vi "ex_subExcelFileWrite.vi"(8 "error in (no error)":errorcluster, 9 "configurations":T1={"new_file"=FALSE, "multi_file"=FALSE, "Enable"=TRUE, "File Dialog"=FALSE, "x_columns"=enum."none", "Ask each iteration"=FALSE, "overwrite_mode"=enum."overwrite", "setting"={"new_file_mode"=1, "Width"=2, "time_format_string"="%Y-%m-%d", "fixed_width"=TRUE, "overwrite_mode_multi"=1, "serno_digits"=3}, "new file options"={{"new_file_iter"=FALSE, "new_file_#iter"=0}, {"new_file_samples"=FALSE, "new_file_#samples"=0}, {"new_file_size"=FALSE, "new_file_max_size"=0}, {"new_file_elaps_time"=FALSE, "seconds"=0}, {"new_file_daily"=FALSE, "new_file_timeofday"=0}}, "reset"=FALSE, "Flush"=FALSE, "Static File Path in"=path "", "timestamp"={"absolute time"=TRUE, "Timestamp format"=""}} {"setting"."new_file_mode" items=["Date & Time", "Serial No.", "Both"]}, 10 "File path":path, 11 "Signals":dynamicdata(waveform)) -> (0 "error out":errorcluster, 2 "Saving Data":bool, 3 "Filename out":path)   [LabVIEW 2020]
uses:
  <vilib>/express/express output/ExFileWriteBlock.llb/ex_ExcelAllConfig.ctl
  <vilib>/express/express output/ExFileWriteBlock.llb/ex_NewFileOptions.ctl
  <vilib>/express/express output/ExFileWriteBlock.llb/ex_ExcelAdvancedConfig.ctl
  <vilib>/express/express shared/ExFile.llb/ex_userDefProperty.ctl
  <vilib>/express/express shared/ex_EditUserDefinedProperties/usiDataType.ctl
  <vilib>/express/express shared/ExFile.llb/ex_propertySource.ctl
  <vilib>/express/express shared/NI_ExcelFile/Ctrls/ExcelRefnum.ctl
  <vilib>/express/express shared/NI_ExcelFile/Ctrls/MainData.ctl
  <vilib>/express/express shared/NI_ExcelFile/Ctrls/StreamMode.ctl
  <vilib>/express/express shared/NI_ExcelFile/Ctrls/TimeColumnMode.ctl
  <vilib>/express/express shared/NI_ExcelFile/Ctrls/FileAttribute.ctl
  <vilib>/express/express shared/NI_ExcelFile/Ctrls/Columns.ctl
  <vilib>/express/express shared/NI_ExcelFile/Ctrls/ColumnInfo.ctl
  <vilib>/express/express shared/NI_ExcelFile/Ctrls/DataType.ctl
  <vilib>/express/express shared/NI_ExcelFile/Ctrls/wd_recordInfo.ctl
  <vilib>/express/express shared/NI_ExcelFile/Ctrls/disk_TemplateFile.ctl
  <vilib>/express/express shared/NI_ExcelFile/Ctrls/meta_file.ctl
  <vilib>/express/express shared/NI_ExcelFile/Ctrls/meta_Block.ctl
  <vilib>/express/express shared/NI_ExcelFile/Ctrls/meta_BlockType.ctl
  <vilib>/express/express shared/NI_ExcelFile/NI_ExcelFile.lvlib
panel:
  out "previous path":path
  in  "1st":bool
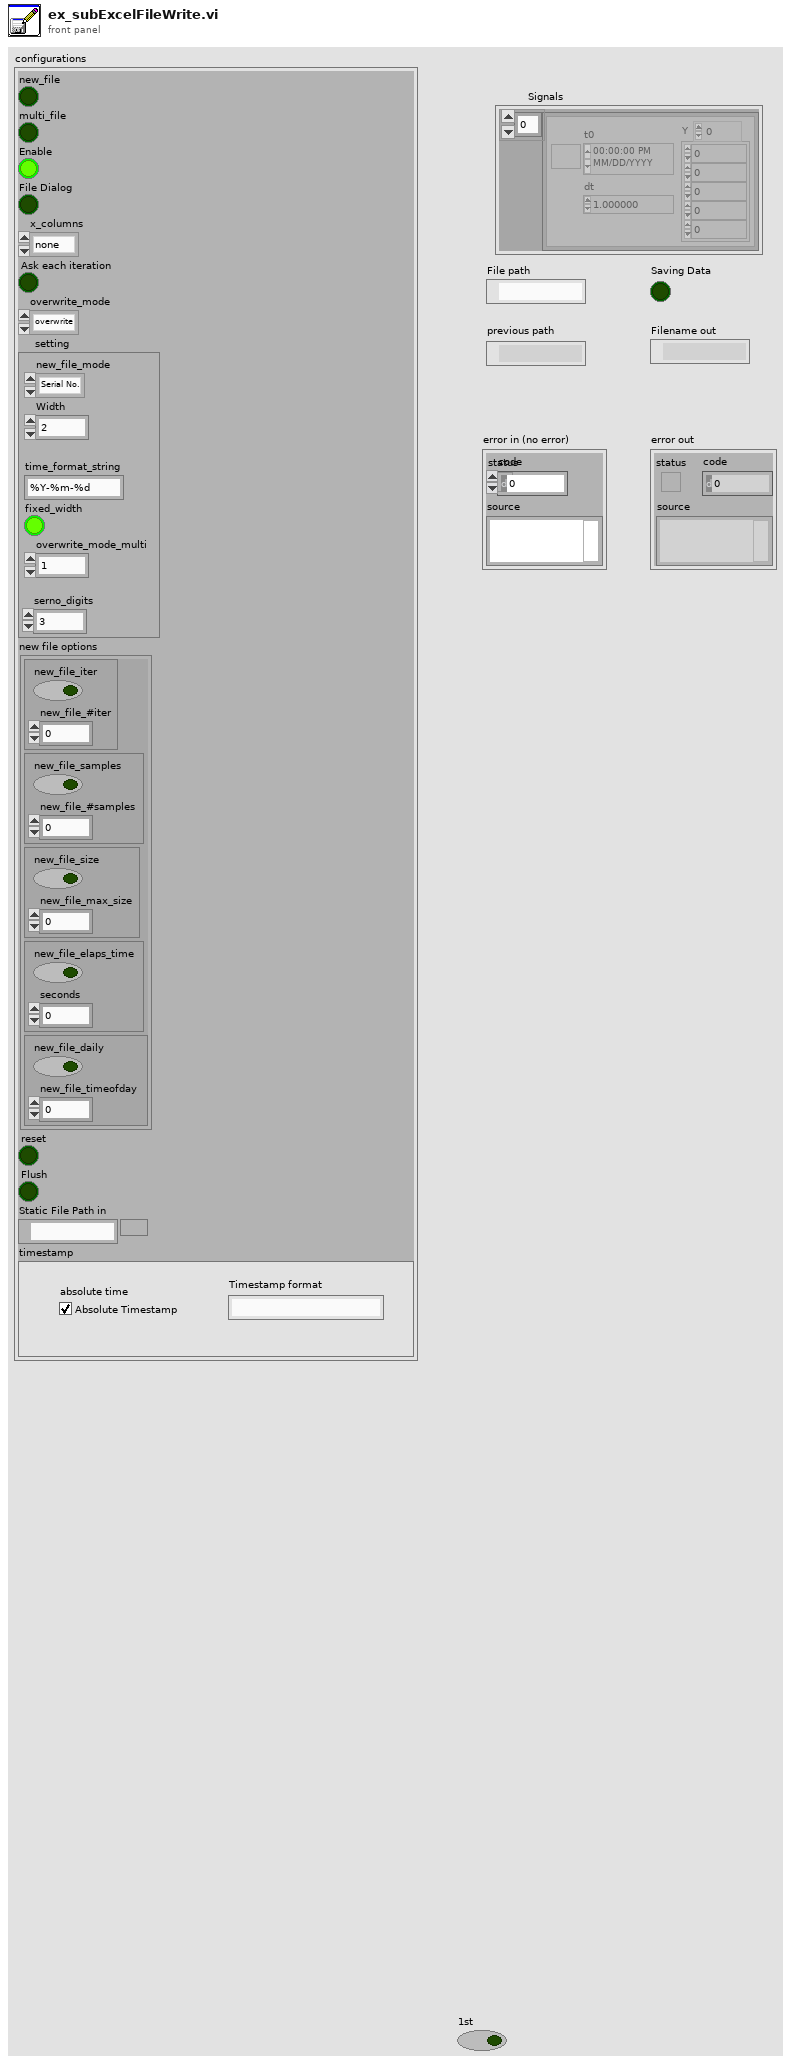
[diagram p1: front panel]
types:
  T1 = typedef "ex_ExcelAllConfig.ctl" = cluster{"new_file":bool, "multi_file":bool, "Enable":bool, "File Dialog":bool, "x_columns":enum32{"none", "one", "multiple"}, "Ask each iteration":bool, "overwrite_mode":enum32{"overwrite", "overwrite & backup", "append", "next avail"}, "setting":cluster{"new_file_mode":u16, "Width":i32, "time_format_string":string, "fixed_width":bool, "overwrite_mode_multi":i32, "serno_digits":i32}, "new file options":T2, "reset":bool, "Flush":bool, "Static File Path in":path, "timestamp":T3}
  T2 = typedef "ex_NewFileOptions.ctl" = cluster{cluster{"new_file_iter":bool, "new_file_#iter":i32}, cluster{"new_file_samples":bool, "new_file_#samples":i32}, cluster{"new_file_size":bool, "new_file_max_size":i32}, cluster{"new_file_elaps_time":bool, "seconds":i32}, cluster{"new_file_daily":bool, "new_file_timeofday":i32}}
  T3 = typedef "ex_ExcelAdvancedConfig.ctl" = cluster{"absolute time":bool, "Timestamp format":string}
  T4 = typedef "ex_userDefProperty.ctl" = cluster{"Name":string, "Object type":string, "usiDataType":T5, "propertySourceType":T6, "propertySource":string, "Value":variant, "ID":i32, "use def name":bool, "Source":string, "Built-in Prop":bool, "Attribute Type Enum":string[]}
  T5 = typedef "usiDataType.ctl" = enum16{"eNoTypeUsi", "eInt8Usi", "eInt16Usi", "eInt32Usi", "eInt64Usi", "eUInt8Usi", "eUInt16Usi", "eUInt32Usi", "eUInt64Usi", "eFloat32Usi", "eFloat64Usi", "- 0", "- 1", "- 2", "- 3", "- 4", "- 5", "- 6", "- 7", "- 8", "- 9", "eString8Usi", "eString16Usi", "eStringUsi", "eEnumUsi", "- 10", "- 11", "- 12", "- 13", "- 14", "eTimeUsi", "- 15", "- 16", "- 17", "- 18", "- 19", "- 20", "- 21", "- 22", "- 23", "eInstanceUsi", "eStoreUsi"}
  T6 = typedef "ex_propertySource.ctl" = enum16{"Manual", "System", "DAQmx Channel", "Terminal", "Ignore"}
  T7 = cluster{"Description":string, "Configure User Def Prop In":cluster{"user-def properties in":T4[]}}
  T8 = typedef "NI_ExcelFile.lvlib/ExcelRefnum.ctl" = refnum<data-value>
  T9 = cluster{"Start Timestamp":timestamp, "Timestamp":timestamp, "Relative Time?":bool, "X Dimension":string, "Signal Name":string, "Y Units":string, "X0":timestamp, "dX":dbl, "nPoints":i32}[]
  T10 = enum32{"overwrite", "overwrite & backup", "append", "next avail"}
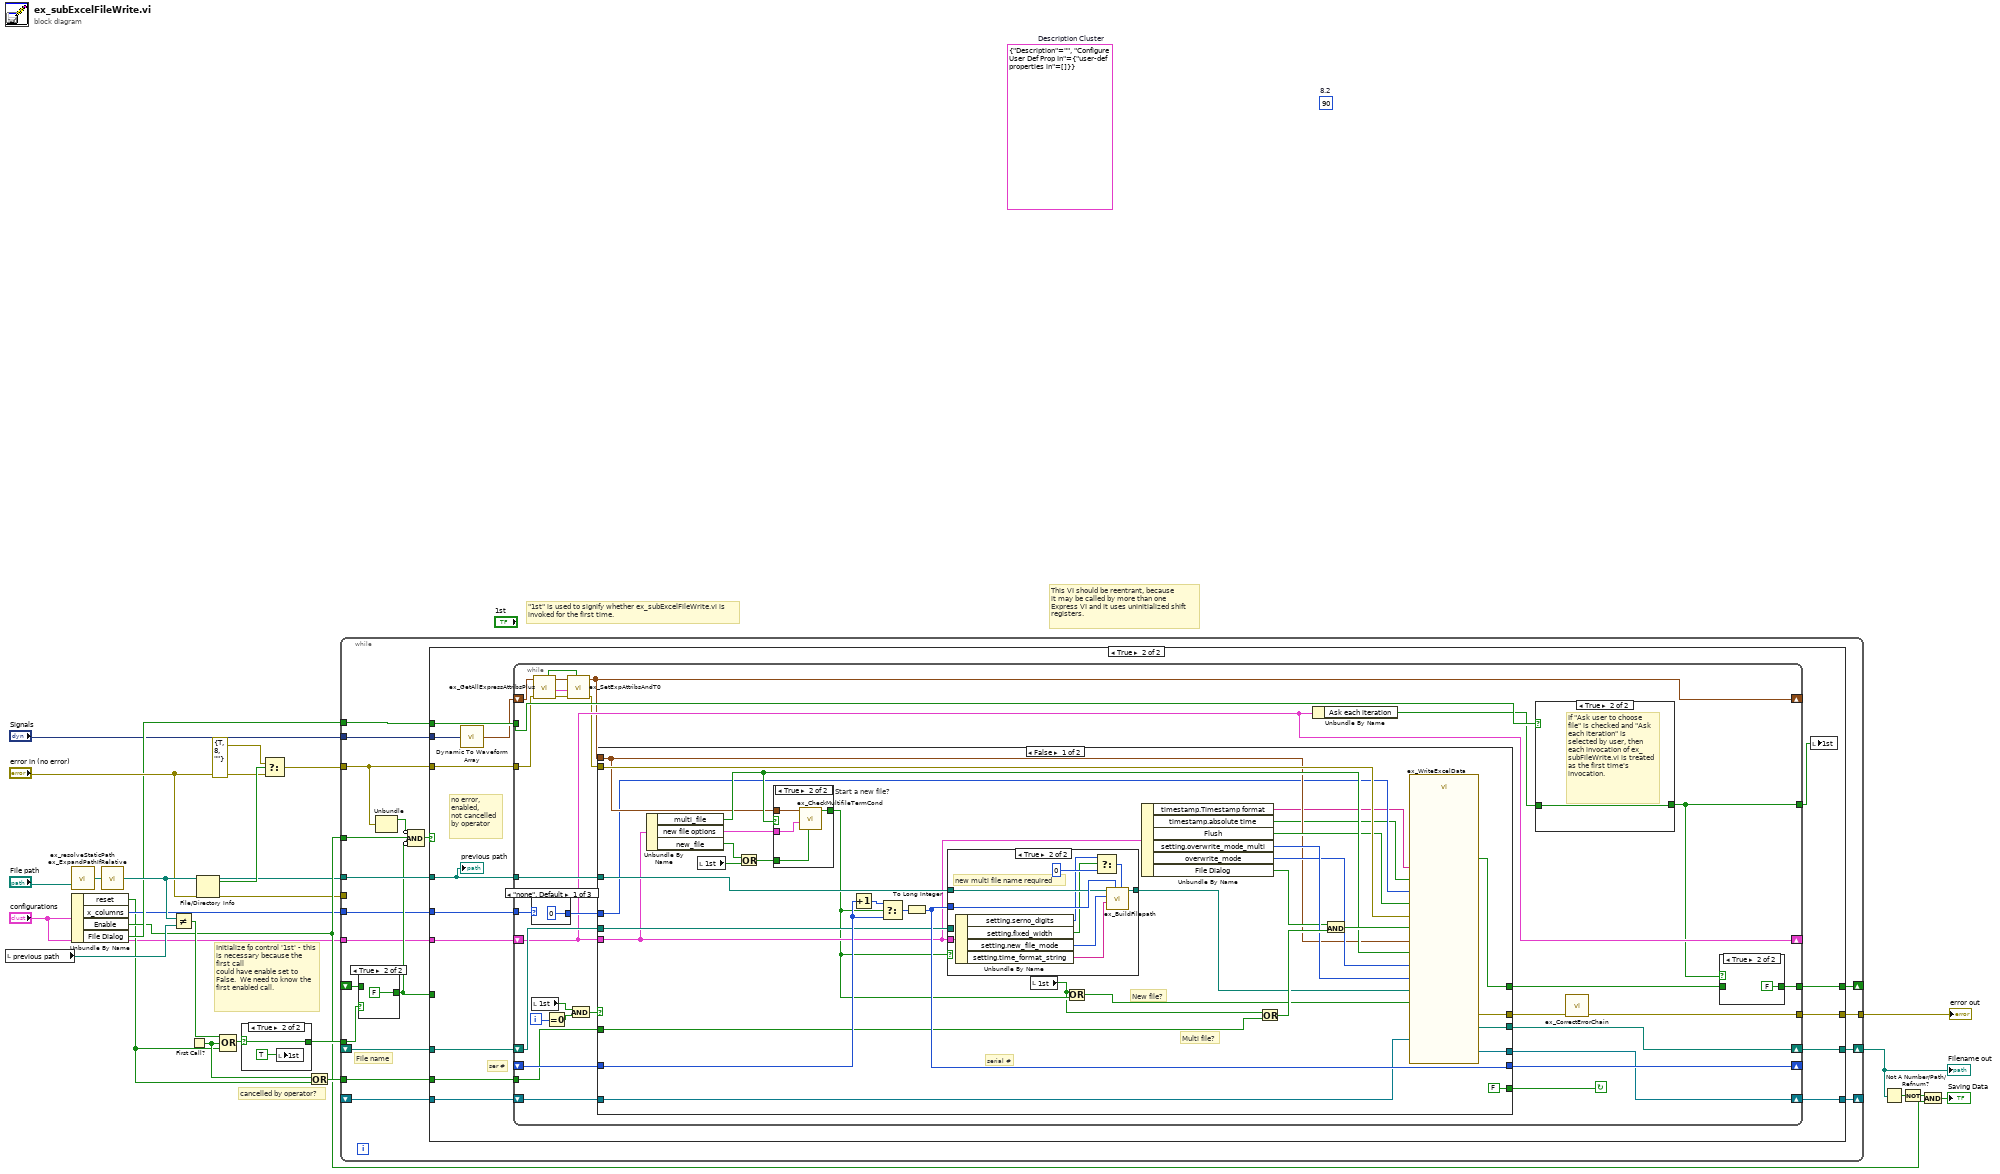
[diagram p0: block diagram]
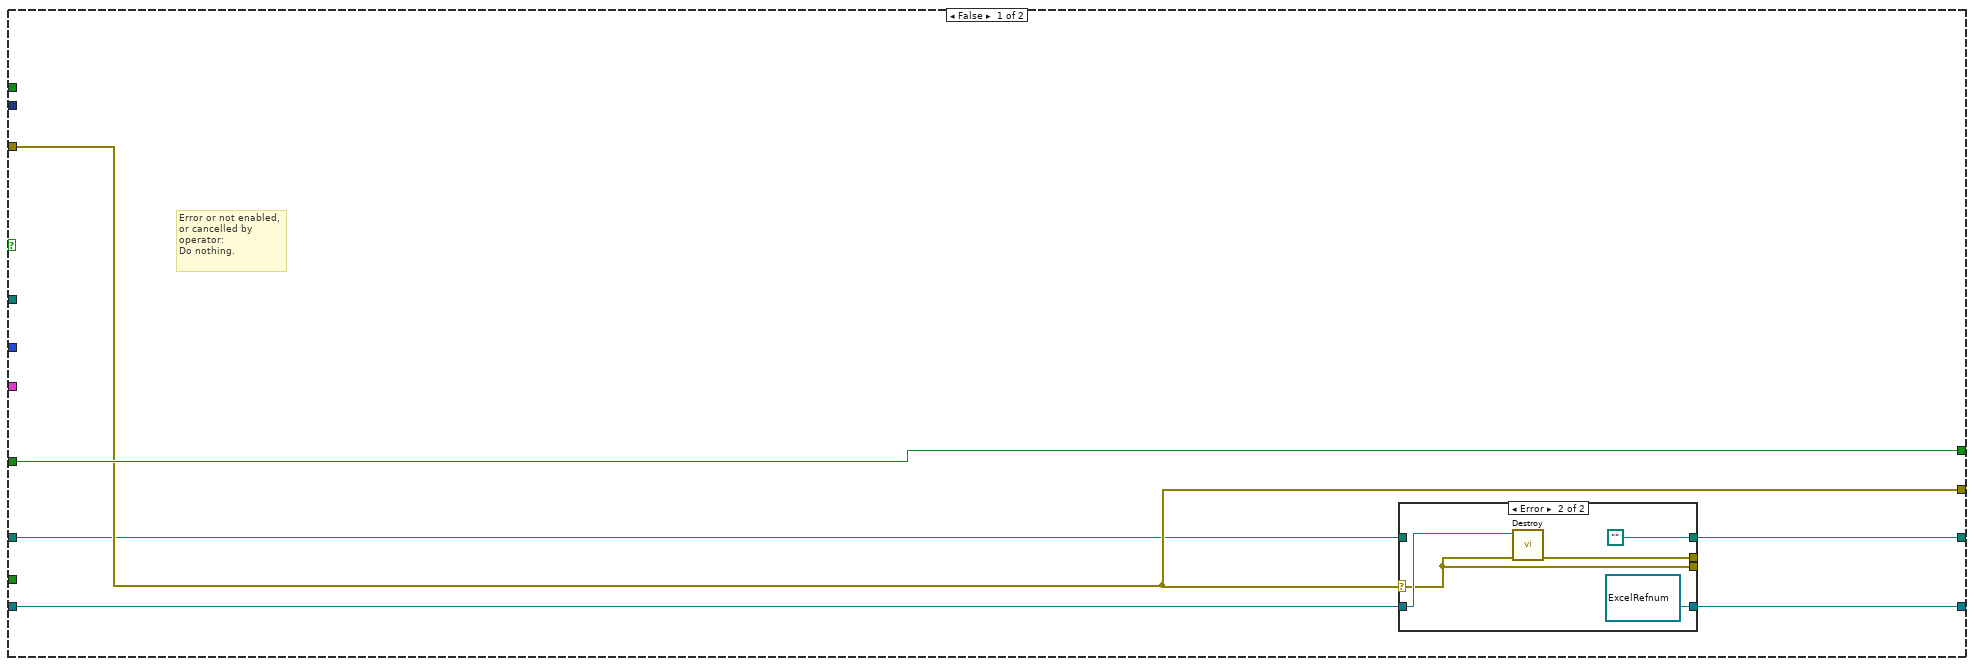
[diagram p3: hidden frame]
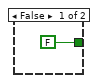
[diagram p7: hidden frame]
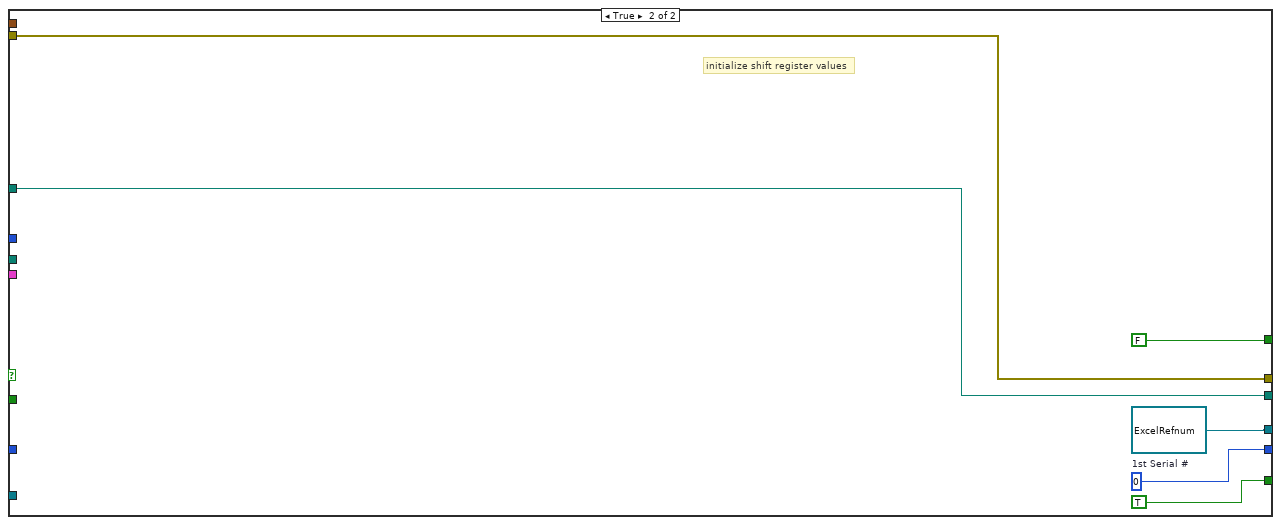
[diagram p8: hidden frame]
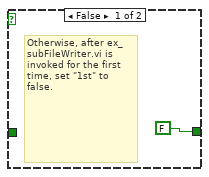
[diagram p9: hidden frame]
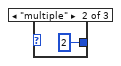
[diagram p10: hidden frame]
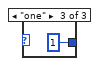
[diagram p11: hidden frame]
diagram:
  (unwired) 90  # 8.2
  (unwired) T7 {"Description"="", "Configure User Def Prop In"={"user-def properties in"=[]}}  # Description Cluster
  # "\"1st\" is used to signify whether ex_subExcelFileWrite.vi is invoked for the first time."
  # "This VI should be reentrant, because\nit may be called by more than one\nExpress VI and it uses uninitialized shift \nregisters."
  # "cancelled by operator?"
  # "Initialize fp control '1st' - this is necessary because the first call\ncould have enable set to False.  We need to know the first enabled call."
  n1 = local read "previous path"() -> (w22:path)
  n2 = call <vilib>:"ex_resolveStaticPath.vi"("file path in"="File path") -> ("Path"=w15:path)  [unwired: 1 in]
  n3 = Unbundle By Name("configurations") -> ("reset"=w5:bool, "x_columns"=w6:enum32{"none", "one", "multiple"}, "Enable"=w8:bool, "File Dialog"=w9:bool)
  n4 = call <vilib>:"ex_ExpandPathIfRelative.vi"("Path"=w15) -> ("Expanded path"=w14:path)  [unwired: 4 out]
  n5 = Not Equal?(x=w14, y=w22) -> (x != y?=w20:bool)
  n6 = First Call?() -> (First Call?: T/F=w19:bool)
  n7 = File/Directory Info(path=w14, error in="error in (no error)") -> (path out=w4:path, directory=w12:bool, error out=w7:errorcluster)  [unwired: 4 out]
  n8 = Compound Arithmetic op=OR(w20, w19, w5) -> (w21:bool)
  n9 = case shown="True" w21 {
    selector: w21 -> [w27 w28]
    tunnel: [w27 w28] -> w26
    frame False {
    }
    frame True {
      n10 = local write "1st"(TRUE ("1st")) -> ()
    }
  }
  n11 = Select(t=errorcluster {"status"=TRUE, "code"=8, "source"=""}, s=w12, f="error in (no error)") -> (s? t:f=w13:errorcluster)
  n12 = Or(x=w19, y=w5) -> (x .or. y?=w18:bool)
  n13 = while {
    tunnel: [w49] -> w17
    tunnel: w26 -> [w35]
    tunnel: w13 -> [w47]
    shift-right: [w45] -> _
    shift-left: _ -> [w44]
    shift-right: [w42] -> w16
    shift-left: _ -> [w43]
    tunnel: w8 -> [w41]
    tunnel: w4 -> [w40]
    tunnel: w18 -> [w37]
    tunnel: "configurations" -> [w36]
    tunnel: w9 -> [w34]
    tunnel: w7 -> [_]
    tunnel: "Signals" -> [w33]
    tunnel: w6 -> [w32]
    shift-right: [w31] -> _
    shift-left: _ -> [w30]
    stop <- FALSE continue-if-true
    # "File name"
    n14 = case shown="True" w35 {
      tunnel: w44 -> [w50 _]
      tunnel: [w50 FALSE ("operator cancelled?")] -> w38
      frame False {
      }
      frame True {
      }
    }
    n15 = Unbundle(w47) -> ("status"=w39:bool)  [unwired: 2 out]
    n16 = Compound Arithmetic op=AND(invert w39, w41, invert w38) -> (w48:bool)
    n17 = case shown="True" w48 {
      tunnel: [w56 w74] -> w49
      tunnel: w47 -> [w56 w80]
      tunnel: [w57 w79] -> w45
      tunnel: w38 -> [w57 _]
      tunnel: [w55 w78] -> w42
      tunnel: w43 -> [w54 w77]
      tunnel: w40 -> [_ w73]
      tunnel: w37 -> [_ w76]
      tunnel: w36 -> [_ w75]
      tunnel: w34 -> [_ w71]
      tunnel: w33 -> [_ w68]
      tunnel: w32 -> [_ w69]
      tunnel: [w53 w66] -> w31
      tunnel: w30 -> [w52 w67]
      frame False {
        # "Error or not enabled,\nor cancelled by\noperator:\nDo nothing."
        n18 = case shown="Error" w56 {
          selector: w56 -> [w58 w61]
          tunnel: [w60 path ""] -> w55
          tunnel: w54 -> [w60 _]
          tunnel: w52 -> [w59 w63]
          tunnel: [w59 T8 refnum ("Excel refnum out")] -> w53
          tunnel: [w58 w61] -> _
          tunnel: [w58 w62] -> _
          frame No Error {
          }
          frame Error {
            n19 = call <vilib>:"Destroy.vi"("error in (no error)"=w61, "Excel refnum"=w63) -> ("error out"=w62:errorcluster)  [unwired: 8 in, 1 out]
          }
        }
      }
      frame True {
        # "no error,\nenabled,\nnot cancelled\nby operator"
        # "ser #"
        n20 = call <vilib>:"Dynamic To Waveform Array.vi"("Input"=w68) -> ("Output"=w70:waveform(dbl)[])  [unwired: 4 out]
        n21 = while {
          tunnel: w80 -> [w86]
          shift-right: [w109] -> _
          shift-left: _ -> [w108]
          tunnel: [w110] -> w74
          shift-right: [w105] -> w78
          shift-left: w77 -> [w107]
          tunnel: w73 -> [w106]
          tunnel: [w81] -> w79
          shift-right: [w84] -> _
          shift-left: w70 -> [w87]
          tunnel: w76 -> [w104]
          shift-right: [w101] -> _
          shift-left: w75 -> [w101]
          tunnel: [w83] -> w72
          tunnel: w71 -> [w102]
          tunnel: w69 -> [w99]
          shift-right: [w97] -> w66
          shift-left: w67 -> [w98]
          i -> [w93]
          stop <- w111 continue-if-true
          n22 = local read "1st"() -> (w94:bool)
          n23 = case shown="\"none\", Default" w99 {
            tunnel: [u16 0 ("x_columns") u16 2 ("x_columns") u16 1 ("x_columns")] -> w103
            frame "none", Default {
            }
            frame "multiple" {
            }
            frame "one" {
            }
          }
          n24 = call <vilib>:"ex_GetAllExpressAttribsPlus.vi"("error in"=w86, "Signals in"=w87) -> ("error out"=w89:errorcluster, "All Express Wave Attributes Plus"=w88:T9, "Signals out"=w91:waveform(dbl)[], "Time Attribs Not Found"=w90:bool[])  [unwired: 1 in, 5 out]
          n25 = Equal To 0?(x=w93) -> (x = 0?=w95:bool)
          n26 = call <vilib>:"ex_SetExpAttribsAndT0.vi"("Set? (T if empty)"=w90, "error in (no error)"=w89, "Express Attributes Plus in"=w88, "Signals"=w91) -> ("error out"=w85:errorcluster, "Signals With Attributes"=w84:waveform(dbl)[])  [unwired: 2 in, 4 out]
          n27 = And(x=w94, y=w95) -> (x .and. y?=w92:bool)
          n28 = case shown="False" w92 {
            tunnel: [FALSE TRUE] -> w111
            tunnel: [w146 w165] -> w109
            tunnel: w108 -> [w145 _]
            tunnel: w107 -> [w144 _]
            tunnel: w106 -> [w143 w168]
            tunnel: [w142 FALSE ("operator cancelled?")] -> w82
            tunnel: [w141 w168] -> w105
            tunnel: w104 -> [w140 _]
            tunnel: w103 -> [w116 _]
            tunnel: w85 -> [w139 w166]
            tunnel: w101 -> [w138 _]
            tunnel: w98 -> [w137 _]
            tunnel: [w136 T8 refnum ("Excel refnum out")] -> w97
            tunnel: w84 -> [w118 _]
            tunnel: [w117 w166] -> w96
            frame False {
              # "Multi file?"
              # "New file?"
              # "serial #"
              n29 = Unbundle By Name(w138) -> ("multi_file"=w123:bool, "new file options"=w126:T2, "new_file"=w122:bool)
              n30 = local read "1st"() -> (w121:bool)
              n31 = Or(x=w122, y=w121) -> (x .or. y?=w120:bool)
              n32 = case "Start a new file?" shown="True" w123 {
                tunnel: [FALSE ("start new file?") w163] -> w133
                tunnel: w126 -> [_ w162]
                tunnel: w120 -> [_ w161]
                tunnel: w118 -> [_ w160]
                frame False {
                }
                frame True {
                  n33 = call <vilib>:"ex_CheckMultifileTermCond.vi"("new_file_now"=w161, "termination conditions"=w162, "Signals"=w160) -> ("start new file?"=w163:bool)  [unwired: 1 in, 7 out]
                }
              }
              n34 = Increment(x=w145) -> (x+1=w135:i32)
              n35 = Select(t=w135, s=w133, f=w145) -> (s? t:f=w134:i32)
              n36 = To Long Integer(number=w134) -> (32bit integer=w146:i32)
              n37 = case shown="True" w133 {
                tunnel: w146 -> [_ w158]
                tunnel: [w148 w157] -> w125
                tunnel: w144 -> [w148 _]
                tunnel: w143 -> [_ w156]
                tunnel: w138 -> [_ w153]
                frame False {
                  # "No new file - use old file name"
                }
                frame True {
                  # "new multi file name required"
                  n38 = Unbundle By Name(w153) -> ("setting.serno_digits"=w152:i32, "setting.fixed_width"=w151:bool, "setting.new_file_mode"=w150:u16, "setting.time_format_string"=w149:string)
                  n39 = Select(t=w152, s=w151, f=0) -> (s? t:f=w154:i32)
                  n40 = call <vilib>:"ex_BuildFilepath.vi"("serial digits"=w154, "serial num"=w158, "time format string"=w149, "naming mode"=w150, "name base"=w156) -> ("built name"=w157:path)  [unwired: 1 in, 5 out]
                }
              }
              n41 = local read "1st"() -> (w130:bool)
              n42 = Or(x=w130, y=w133) -> (x .or. y?=w124:bool)
              n43 = Unbundle By Name(w138) -> ("timestamp.Timestamp format"=w115:string, "timestamp.absolute time"=w114:bool, "Flush"=w119:bool, "setting.overwrite_mode_multi"=w129:i32, "overwrite_mode"=w128:T10, "File Dialog"=w127:bool)
              n44 = Or(x=w130, y=w140) -> (x .or. y?=w132:bool)
              n45 = And(x=w127, y=w132) -> (x .and. y?=w131:bool)
              n46 = call <vilib>:"ex_WriteExcelData.vi"("file path"=w125, "Signals"=w118, "Excel refnum"=w137, "absolulte time (yes:T)"=w114, "overwrite_mode_multi"=w129, "overwrite_mode"=w128, "x_columns"=w116, "error in (no error)"=w139, "file dialog?"=w131, "Flush"=w119, "timestamp format"=w115, "multi_file"=w123, "new file?"=w124) -> ("operator cancelled?"=w142:bool, "file path out"=w141:path, "Excel refnum out"=w136:T8, "error out"=w117:errorcluster)  [unwired: 11 in]
            }
            frame True {
              w165 = 0  # 1st Serial #
              # "initialize shift register values"
            }
          }
          n47 = Unbundle By Name(w101) -> ("Ask each iteration"=w100:bool)
          n48 = case shown="True" w102 {
            tunnel: [FALSE ("Ask each iteration") w171] -> w83
            tunnel: w100 -> [_ w171]
            frame False {
              # "Otherwise, after ex_subFileWriter.vi is invoked for the first time, set \"1st\" to false."
            }
            frame True {
              # "If \"Ask user to choose file\" is checked and \"Ask each iteration\" is selected by user, then each invocation of ex_subFileWrite.vi is treated as the first time's invocation."
            }
          }
          n49 = call <vilib>:"ex_CorrectErrorChain.vi"("error in (no error)"=w96) -> ("error out"=w110:errorcluster)  [unwired: 1 in, 9 out]
          n50 = case shown="True" w83 {
            tunnel: w82 -> [w112 _]
            tunnel: [w112 FALSE ("operator cancelled?")] -> w81
            frame False {
            }
            frame True {
            }
          }
        }
        n51 = local write "1st"(w72) -> ()
        "previous path" <- w73
      }
    }
  }
  "error out" <- w17
  "Filename out" <- w16
  n52 = Not A Number/Path/Refnum?(number/path/refnum=w16) -> (NaN/Path/Refnum?=w25:bool)
  n53 = Not(x=w25) -> (.not. x?=w24:bool)
  n54 = And(x=w24, y=w8) -> (x .and. y?=→"Saving Data":bool)
